vi "Rectangular Target - 2013 (2).vi"(2 "acc":dbl, 3 "Yinput":dbl, 4 "Xinput":dbl) -> (0 "Youtput":dbl format="%.2f", 1 "Xoutput":dbl format="%.2f")   [LabVIEW 2012]
uses:
  <vilib>/addons/control/pid/pid.llb/PID Output Rate Limiter (DBL).vi
  <vilib>/addons/control/pid/pid.llb/PID Control Input Filter (DBL).vi
  <vilib>/addons/control/pid/NI_PID_pid.lvlib
  <vilib>/addons/control/pid/pid.llb/PID Lead-Lag (DBL).vi
panel:
  in  "fNode":dbl
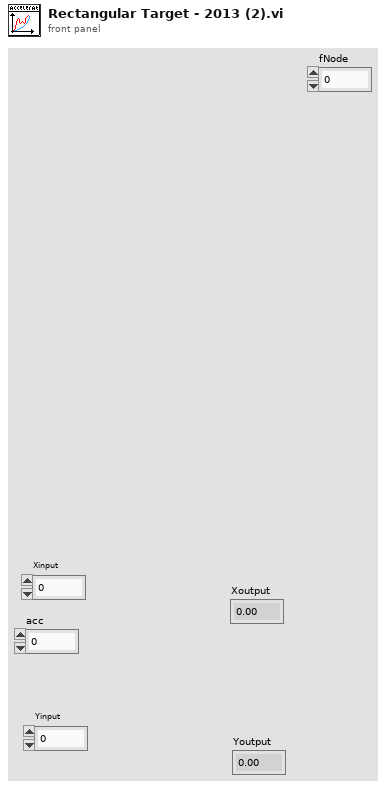
[diagram p1: front panel]
types:
  T1 = cluster{"gain":dbl, "lag time (min)":dbl, "lead time (min)":dbl}
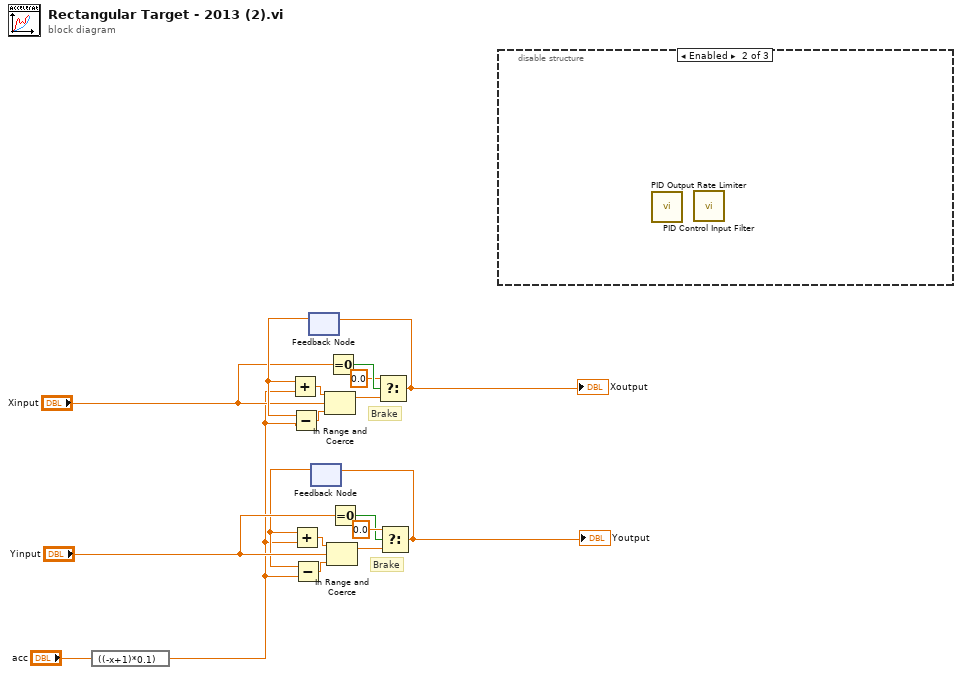
[diagram p0: block diagram]
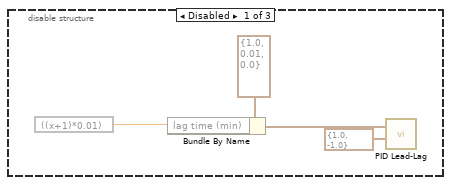
[diagram p2: hidden frame]
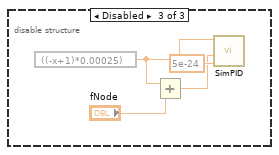
[diagram p3: hidden frame]
diagram:
  # "Brake"
  # "Brake"
  n1 = expression code="((-x+1)*0.1)"("acc") -> (w1:dbl)
  n2 = feedback #1() -> (w16:dbl)  [unwired: 1 in]
  n3 = Add(x=w16, y=w1) -> (x+y=w17:dbl)
  n4 = Subtract(x=w16, y=w1) -> (x-y=w18:dbl)
  n5 = feedback #2() -> (w4:dbl)  [unwired: 1 in]
  n6 = Add(x=w4, y=w1) -> (x+y=w3:dbl)
  n7 = Subtract(x=w4, y=w1) -> (x-y=w2:dbl)
  n8 = In Range and Coerce(upper limit=w17, x="Xinput", lower limit=w18) -> (coerced(x)=w12:dbl)  [unwired: 1 out]
  n9 = In Range and Coerce(upper limit=w3, x="Yinput", lower limit=w2) -> (coerced(x)=w7:dbl)  [unwired: 1 out]
  n10 = Equal To 0?(x="Xinput") -> (x = 0?=w13:bool)
  n11 = Equal To 0?(x="Yinput") -> (x = 0?=w6:bool)
  n12 = Select(t=0.0, s=w13, f=w12) -> (s? t:f=w10:dbl)
  "Xoutput" <- w10
  n13 = feedback-in #1(w10) -> ()
  n14 = Select(t=0.0, s=w6, f=w7) -> (s? t:f=w9:dbl)
  "Youtput" <- w9
  n15 = feedback-in #2(w9) -> ()
  n16 = disable-structure shown="Enabled" {
    frame Disabled {
      n17 = expression code="((x+1)*0.01)"() -> (w23:dbl)  [unwired: 1 in]
      n18 = Bundle By Name(cluster=T1 {"gain"=1.0, "lag time (min)"=0.01, "lead time (min)"=0.0} ("tuning parameters"), "lag time (min)"=w23) -> (w22:T1)
      n19 = call-poly <vilib>:"PID Lead-Lag.vi"("output range"=cluster{"output high":dbl, "output low":dbl} {"output high"=1.0, "output low"=-1.0}, "tuning parameters"=w22) -> ("output"=w20:dbl, "reinitialize? (F)"=w21:bool, "input"=w19:dbl)  [unwired: 2 in, 3 out]
    }
    frame Enabled {
      n20 = call-poly <vilib>:"PID Output Rate Limiter.vi"() -> ()  [unwired: 8 in, 2 out]
      n21 = call-poly <vilib>:"PID Control Input Filter.vi"() -> ()  [unwired: 5 in, 1 out]
    }
    frame Disabled {
      n22 = expression code="((-x+1)*0.00025)"() -> (w28:dbl)  [unwired: 1 in]
      n23 = Add(x=w28, y="fNode") -> (x+y=w27:dbl)
      n24 = call "SimPID.vi"("Range"=5e-24, "Position"=w27, "Gain"=w28) -> ("result"=w29:dbl, "Set Point"=w30:dbl)  [unwired: 5 in, 1 out]
    }
  }
